vi "Verify Remote Repository.vi"(8 "error in (no error)":errorcluster, 10 "folder (root)":string, 11 "Artifactory in":refnum<class "Artifactory.lvclass">) -> (0 "error out":errorcluster, 1 "Read Permissions":bool, 2 "Repository exists":bool, 3 "Artifactory out":refnum<class "Artifactory.lvclass">)   [LabVIEW 2021, in "Artifactory.lvclass"]
uses:
  Artifactory.lvclass
  Artifactory.lvclass/Artifactory.ctl
  Actions -- enum.ctl
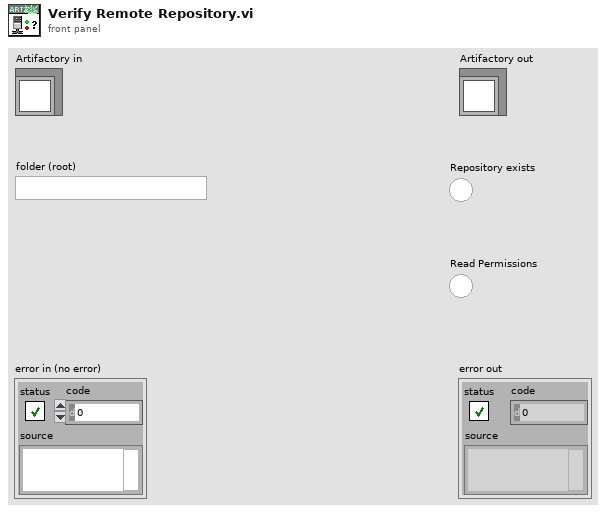
[diagram p1: front panel]
types:
  T1 = typedef "Artifactory.lvclass/Actions -- enum.ctl" = enum16{"Idle", "Custom Event", "Connecting to Artifactory", "Verifying Permissions", "Listing local repository", "Listing remote repository", "Computing changes", "Uploading file", "Downloading file"}
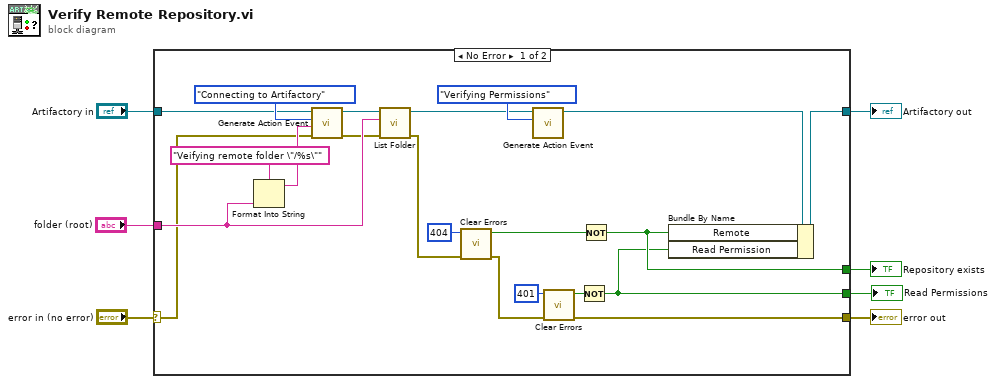
[diagram p0: block diagram]
diagram:
  n1 = case shown="No Error" "error in (no error)" {
    selector: "error in (no error)" -> [w9 w30]
    tunnel: [w21 w30] -> w6
    tunnel: [w26 w29] -> w4
    tunnel: "Artifactory in" -> [w16 w29]
    tunnel: [w23 _] -> w3
    tunnel: "folder (root)" -> [w15 _]
    tunnel: [w22 _] -> w1
    frame No Error {
      n2 = Format Into String(format string="Veifying remote folder \"/%s\"", w15) -> (resulting string=w14:string)  [unwired: 2 in, 1 out]
      n3 = call-dynamic "Generate Action Event.vi"("error in (no error)"=w9, "Description"=w14, "Action"=Actions_--_enum."Connecting to Artifactory", "Artifactory in"=w16) -> ("error out"=w8:errorcluster, "Artifactory out"=w17:refnum<class "Artifactory.lvclass">)  [unwired: 6 in]
      n4 = call "List Folder.vi"("error in (no error)"=w8, "folder (root)"=w15, "Artifactory in"=w17) -> ("error out"=w20:errorcluster, "Artifactory out"=w11:refnum<class "Artifactory.lvclass">)  [unwired: 5 in, 2 out]
      n5 = call <vilib>:"Clear Errors.vi"("error in (no error)"=w20, "specific error code to clear (0: all)"=404) -> ("error out"=w19:errorcluster, "specific error cleared?"=w27:bool)  [unwired: 4 in]
      n6 = call-dynamic "Generate Action Event.vi"("Action"=Actions_--_enum."Verifying Permissions", "Artifactory in"=w11) -> ("Artifactory out"=w10:refnum<class "Artifactory.lvclass">)  [unwired: 8 in, 1 out]
      n7 = call <vilib>:"Clear Errors.vi"("error in (no error)"=w19, "specific error code to clear (0: all)"=401) -> ("error out"=w21:errorcluster, "specific error cleared?"=w24:bool)  [unwired: 4 in]
      n8 = Not(x=w24) -> (.not. x?=w22:bool)
      n9 = Not(x=w27) -> (.not. x?=w23:bool)
      n10 = Bundle By Name(cluster=w10, "Remote"=w23, "Read Permission"=w22) -> (w26:refnum<class "Artifactory.lvclass">)
    }
    frame Error {
    }
  }
  "error out" <- w6
  "Artifactory out" <- w4
  "Repository exists" <- w3
  "Read Permissions" <- w1
